vi "Destroy.vi"(8 "error in (no error)":errorcluster, 11 "Store in":refnum<class "Store.lvclass">) -> (0 "error out":errorcluster)   [LabVIEW 2018, in "Application.lvlib" / "Store.lvclass"]
uses:
  Store.lvclass
  Store.lvclass/Store.ctl
  Dictionary Class/Dictionary.lvclass
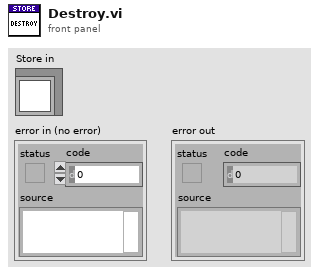
[diagram p1: front panel]
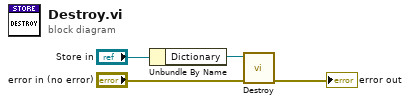
[diagram p0: block diagram]
diagram:
  n1 = Unbundle By Name("Store in") -> ("Dictionary"=w3:refnum<class "Dictionary.lvclass">)
  n2 = call "Destroy.vi"("error in (no error)"="error in (no error)", "Dictionary in"=w3) -> ("error out"=→"error out":errorcluster)  [unwired: 7 in, 2 out]
